vi "main.vi"() -> ()   [LabVIEW 2015]
uses:
  <vilib>/Platform/browser.llb/Open URL in Default Browser (string).vi
  <vilib>/Utility/cursorutil.llb/Set Cursor (Icon Pict).vi
panel:
  in  "VI引用":refnum<vi>
  out "字符串 2":string
  out "字符串":string
  in  "选项卡控件":T1(tab)
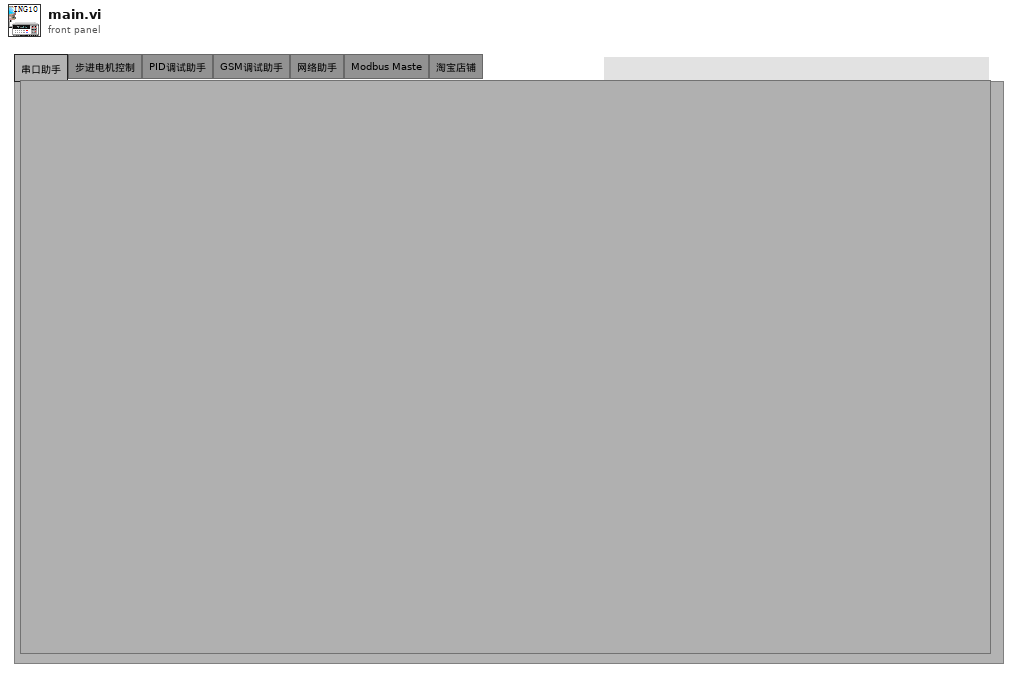
[diagram p1: front panel]
types:
  T1 = enum32{"串口助手", "步进电机控制", "PID调试助手", "GSM调试助手", "网络助手", "Modbus Maste", "淘宝店铺"}
  T2 = typedef "LVPointTypeDef.ctl" = cluster{"Horizontal":i16, "Vertical":i16}
  T3 = typedef "LVRectTypeDef.ctl" = cluster{"Left":i16, "Top":i16, "Right":i16, "Bottom":i16}
  T4 = typedef "LVBoundsTypeDef.ctl" = cluster{"Width":u32, "Height":u32}
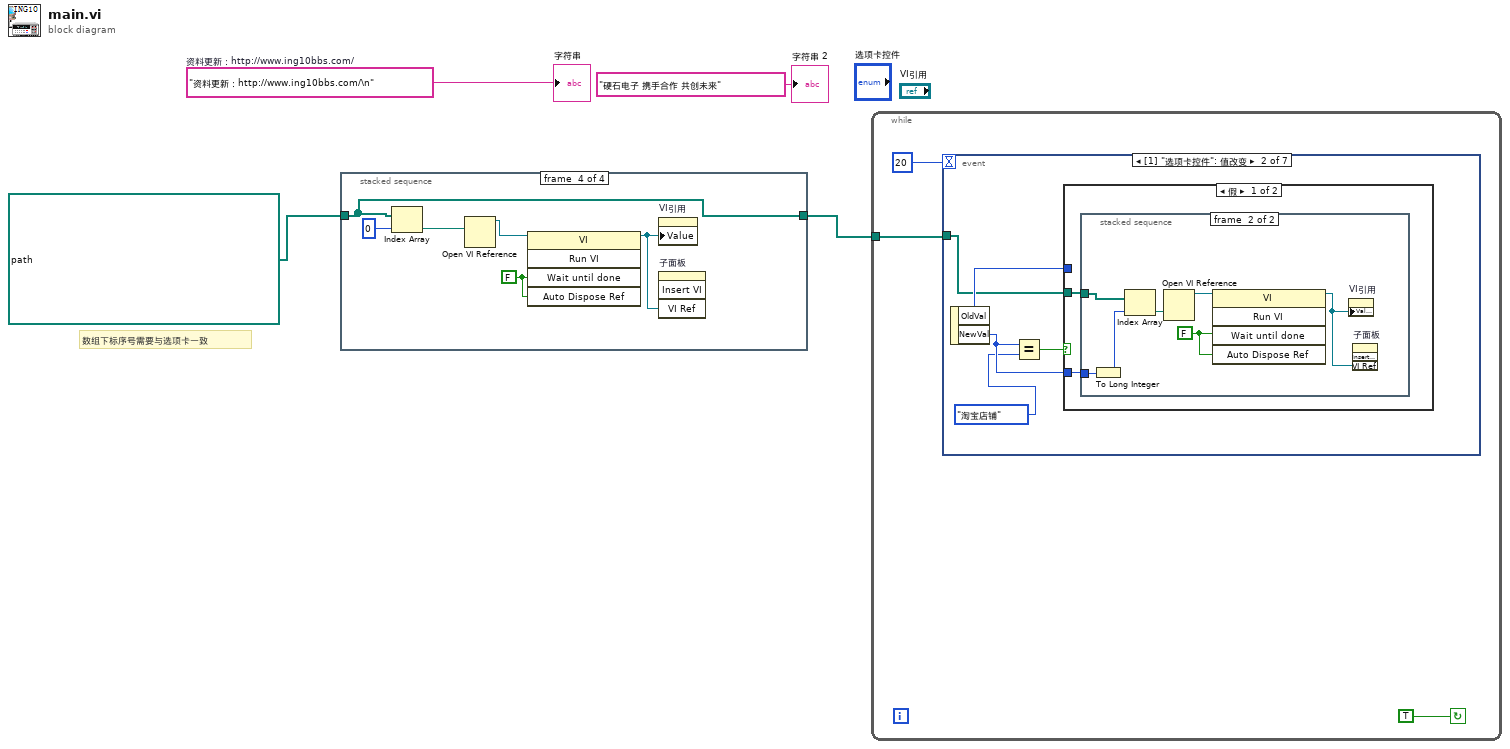
[diagram p0: block diagram]
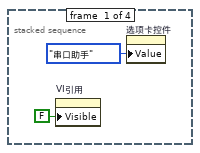
[diagram p2: hidden frame]
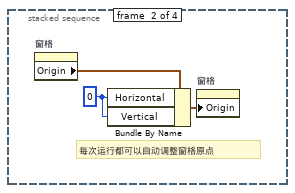
[diagram p3: hidden frame]
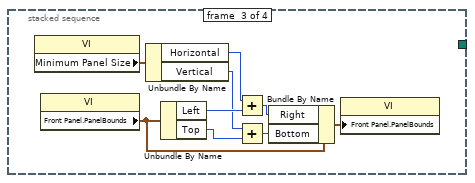
[diagram p4: hidden frame]
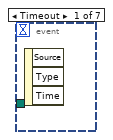
[diagram p5: hidden frame]
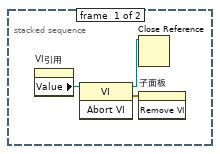
[diagram p6: hidden frame]
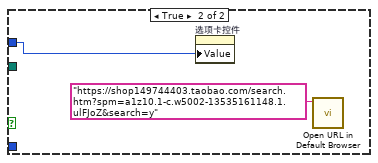
[diagram p7: hidden frame]
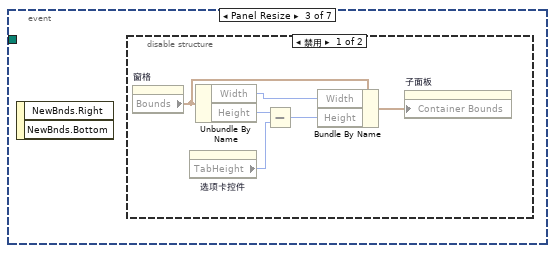
[diagram p8: hidden frame]
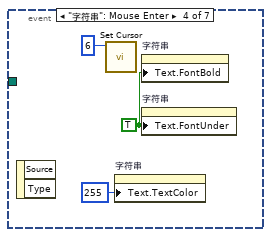
[diagram p10: hidden frame]
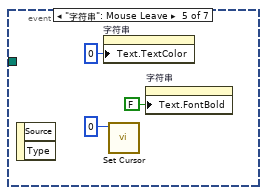
[diagram p11: hidden frame]
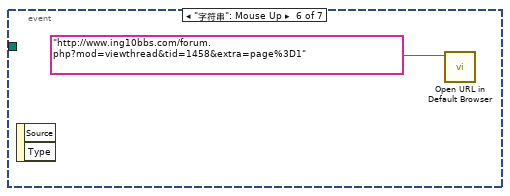
[diagram p12: hidden frame]
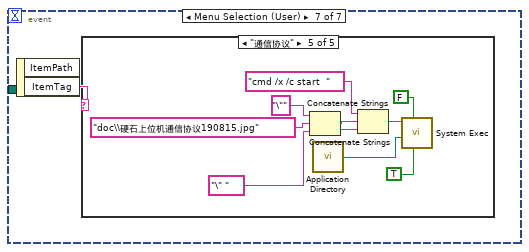
[diagram p13: hidden frame]
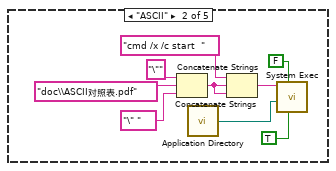
[diagram p15: hidden frame]
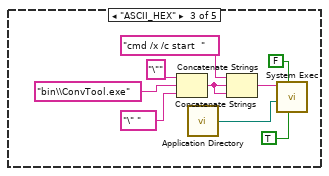
[diagram p16: hidden frame]
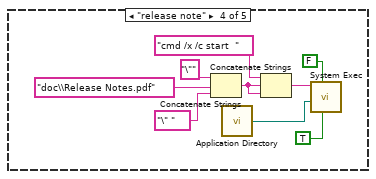
[diagram p17: hidden frame]
diagram:
  w3 = "资料更新：http://www.ing10bbs.com/\n"  # 资料更新：http://www.ing10bbs.com/
  # "数组下标序号需要与选项卡一致"
  n1 = stacked-sequence {
    tunnel: path[] [path "SubVI/串口助手/串口助手.vi", path "SubVI/步进电机控制/步进电机控制.vi", path "SubVI/PID调试助手/PIDdebuger.vi", path "SubVI/GSM调试/GSM调试.vi", path "SubVI/网络通信助手/网络通信.vi", path "SubVI/Modbus调试助手/MB_Master.vi"] -> [_ _ _ w19]
    tunnel: [_ _ _ w19] -> w1
    frame #0 {
      n2 = property on="VI引用" class="VIRef (严格)"("Visible"=FALSE) -> ()  [unwired: 2 in, 2 out]
      n3 = property on="选项卡控件" class="TabCtl (严格)"("Value"=enum16{"串口助手"}."串口助手") -> ()  [unwired: 2 in, 2 out]
    }
    frame #1 {
      w7 = 0
      # "每次运行都可以自动调整窗格原点"
      n4 = property on="窗格" class="Pane"() -> ("Origin"=w8:T2)  [unwired: 2 in, 2 out]
      n5 = Bundle By Name(cluster=w8, "Horizontal"=w7, "Vertical"=w7) -> (w9:T2)
      n6 = property on="窗格" class="Pane"("Origin"=w9) -> ()  [unwired: 2 in, 2 out]
    }
    frame #2 {
      n7 = property class="VI"() -> ("Minimum Panel Size"=w11:T2)  [unwired: 2 in, 2 out]
      n8 = property class="VI"() -> ("Front Panel.PanelBounds"=w10:T3)  [unwired: 2 in, 2 out]
      n9 = Unbundle By Name(w11) -> ("Horizontal"=w16:i16, "Vertical"=w14:i16)
      n10 = Unbundle By Name(w10) -> ("Left"=w17:i16, "Top"=w13:i16)
      n11 = Add(x=w16, y=w17) -> (x+y=w15:i16)
      n12 = Add(x=w14, y=w13) -> (x+y=w12:i16)
      n13 = Bundle By Name(cluster=w10, "Right"=w15, "Bottom"=w12) -> (w18:T3)
      n14 = property class="VI"("Front Panel.PanelBounds"=w18) -> ()  [unwired: 2 in, 2 out]
    }
    frame #3 {
      w20 = FALSE
      n15 = Index Array(array=w19, index=0) -> (element=w21:path)
      n16 = Open VI Reference(vi path=w21) -> (vi reference=w23:refnum<vi>)  [unwired: 5 in, 1 out]
      n17 = invoke class="VI" method="Run VI"(reference=w23, "Wait until done"=w20, "Auto Dispose Ref"=w20) -> (reference out=w24:refnum<vi>)  [unwired: 2 in, 4 out]
      n18 = property on="VI引用" class="VIRef (严格)"("Value"=w24) -> ()  [unwired: 2 in, 2 out]
      n19 = invoke on="子面板" class="子面板" method="Insert VI"("VI Ref"=w24) -> ()  [unwired: 3 in, 4 out]
    }
  }
  n20 = while {
    tunnel: w1 -> [w25]
    stop <- TRUE continue-if-true
    n21 = event shown="[1] \"选项卡控件\": 值改变" {
      selector: _ -> [_ _ _ _ _ _ _]
      dyn-events: _ -> [_ _ _ _ _ _ _]
      timeout: 20 -> [_ _ _ _ _ _ _]
      tunnel: w25 -> [_ w31 _ _ _ _ _]
      event Timeout {
        n22 = event-data() -> ()  [unwired: 1 in, 3 out]
      }
      event "选项卡控件": Value Change {
        n23 = event-data() -> ("OldVal"=w32:T1, "NewVal"=w29:T1)  [unwired: 1 in]
        n24 = Equal?(x=w29, y=T1."淘宝店铺" ("选项卡控件")) -> (x = y?=w30:bool)
        n25 = case shown="假" w30 {
          tunnel: w32 -> [_ w45]
          tunnel: w31 -> [w34 _]
          tunnel: w29 -> [w33 _]
          frame False {
            n26 = stacked-sequence {
              tunnel: w33 -> [_ w44]
              tunnel: w34 -> [_ w43]
              frame #0 {
                n27 = property on="VI引用" class="VIRef (严格)"() -> ("Value"=w35:refnum<vi>)  [unwired: 2 in, 2 out]
                n28 = invoke class="VI" method="Abort VI"(reference=w35) -> (reference out=w36:refnum<vi>, error out=w37:errorcluster)  [unwired: 2 in, 1 out]
                n29 = Close Reference(reference=w36) -> ()  [unwired: 1 in, 1 out]
                n30 = invoke on="子面板" class="子面板" method="Remove VI"(error in=w37) -> ()  [unwired: 2 in, 3 out]
              }
              frame #1 {
                w41 = FALSE
                n31 = To Long Integer(number=w44) -> (32bit integer=w38:i32)
                n32 = Index Array(array=w43, index=w38) -> (element=w40:path)
                n33 = Open VI Reference(vi path=w40) -> (vi reference=w42:refnum<vi>)  [unwired: 5 in, 1 out]
                n34 = invoke class="VI" method="Run VI"(reference=w42, "Wait until done"=w41, "Auto Dispose Ref"=w41) -> (reference out=w39:refnum<vi>)  [unwired: 2 in, 4 out]
                n35 = property on="VI引用" class="VIRef (严格)"("Value"=w39) -> ()  [unwired: 2 in, 2 out]
                n36 = invoke on="子面板" class="SubPnl" method="Insert VI"("VI Ref"=w39) -> ()  [unwired: 3 in, 4 out]
              }
            }
          }
          frame True {
            n37 = property on="选项卡控件" class="TabCtl (严格)"("Value"=w45) -> ()  [unwired: 2 in, 2 out]
            n38 = call-poly <vilib>:"Open URL in Default Browser.vi"("URL"="https://shop149744403.taobao.com/search.htm?spm=a1z10.1-c.w5002-13535161148.1.ulFJoZ&search=y") -> ()  [unwired: 5 in, 2 out]
          }
        }
      }
      event Panel Resize {
        n39 = event-data() -> ()  [unwired: 1 in, 2 out]
        n40 = disable-structure shown="禁用" {
          frame Disabled {
            n41 = property on="窗格" class="Pane"() -> ("Bounds"=w49:T4)  [unwired: 2 in, 2 out]
            n42 = property on="选项卡控件" class="TabCtl (严格)"() -> ("TabHeight"=w52:u32)  [unwired: 2 in, 2 out]
            n43 = Unbundle By Name(w49) -> ("Width"=w48:u32, "Height"=w50:u32)
            n44 = Subtract(x=w50, y=w52) -> (x-y=w47:u32)
            n45 = Bundle By Name(cluster=w49, "Width"=w48, "Height"=w47) -> (w51:T4)
            n46 = property on="子面板" class="SubPnl"("Container Bounds"=w51) -> ()  [unwired: 2 in, 2 out]
          }
          frame Enabled {
          }
        }
      }
      event "字符串": Mouse Enter {
        w53 = TRUE
        n47 = event-data() -> ()  [unwired: 1 in, 2 out]
        n48 = call-poly <vilib>:"Set Cursor.vi"("icon"=u16 6) -> ()  [unwired: 9 in, 2 out]
        n49 = property on="字符串" class="Str"("Text.TextColor"=u32 255) -> ()  [unwired: 2 in, 2 out]
        n50 = property on="字符串" class="Str"("Text.FontBold"=w53) -> ()  [unwired: 2 in, 2 out]
        n51 = property on="字符串" class="Str"("Text.FontUnder"=w53) -> ()  [unwired: 2 in, 2 out]
      }
      event "字符串": Mouse Leave {
        n52 = event-data() -> ()  [unwired: 1 in, 2 out]
        n53 = property on="字符串" class="Str"("Text.TextColor"=u32 0) -> ()  [unwired: 2 in, 2 out]
        n54 = call-poly <vilib>:"Set Cursor.vi"("icon"=u16 0) -> ()  [unwired: 9 in, 2 out]
        n55 = property on="字符串" class="Str"("Text.FontBold"=FALSE) -> ()  [unwired: 2 in, 2 out]
      }
      event "字符串": Mouse Up {
        n56 = event-data() -> ()  [unwired: 1 in, 2 out]
        n57 = call-poly <vilib>:"Open URL in Default Browser.vi"("URL"="http://www.ing10bbs.com/forum.php?mod=viewthread&tid=1458&extra=page%3D1") -> ()  [unwired: 5 in, 2 out]
      }
      event Menu Selection (User) {
        n58 = event-data() -> ("ItemTag"=w60:string)  [unwired: 1 in, 1 out]
        n59 = case shown="\"通信协议\"" w60 {
          frame Default {
          }
          frame "ASCII" {
            n60 = Concatenate Strings("\"" ("Substring"), "doc\\ASCII对照表.pdf", "\" " ("Substring")) -> (w66:string)
            n61 = call <vilib>:"Application Directory.vi"() -> ("Application Directory"=w61:path)
            n62 = Concatenate Strings("cmd /x /c start  ", w66, w66) -> (w68:string)
            n63 = call <vilib>:"System Exec.vi"("run minimized? (F)"=TRUE, "wait until completion? (T)"=FALSE ("Wait until done"), "working directory"=w61, "command line"=w68) -> ()  [unwired: 2 in, 6 out]
          }
          frame "ASCII_HEX" {
            n64 = Concatenate Strings("\"" ("Substring"), "bin\\ConvTool.exe", "\" " ("Substring")) -> (w75:string)
            n65 = call <vilib>:"Application Directory.vi"() -> ("Application Directory"=w70:path)
            n66 = Concatenate Strings("cmd /x /c start  ", w75, w75) -> (w77:string)
            n67 = call <vilib>:"System Exec.vi"("run minimized? (F)"=TRUE, "wait until completion? (T)"=FALSE ("Wait until done"), "working directory"=w70, "command line"=w77) -> ()  [unwired: 2 in, 6 out]
          }
          frame "release note" {
            n68 = Concatenate Strings("\"" ("Substring"), "doc\\Release Notes.pdf", "\" " ("Substring")) -> (w84:string)
            n69 = call <vilib>:"Application Directory.vi"() -> ("Application Directory"=w79:path)
            n70 = Concatenate Strings("cmd /x /c start  ", w84, w84) -> (w86:string)
            n71 = call <vilib>:"System Exec.vi"("run minimized? (F)"=TRUE, "wait until completion? (T)"=FALSE ("Wait until done"), "working directory"=w79, "command line"=w86) -> ()  [unwired: 2 in, 6 out]
          }
          frame "通信协议" {
            n72 = Concatenate Strings("\"" ("Substring"), "doc\\硬石上位机通信协议190815.jpg", "\" " ("Substring")) -> (w93:string)
            n73 = call <vilib>:"Application Directory.vi"() -> ("Application Directory"=w88:path)
            n74 = Concatenate Strings("cmd /x /c start  ", w93, w93) -> (w95:string)
            n75 = call <vilib>:"System Exec.vi"("run minimized? (F)"=TRUE, "wait until completion? (T)"=FALSE ("Wait until done"), "working directory"=w88, "command line"=w95) -> ()  [unwired: 2 in, 6 out]
          }
        }
      }
    }
  }
  "字符串 2" <- "硬石电子 携手合作 共创未来"
  "字符串" <- w3
